vi "SetOscillatorFreq.vi"(8 "error in (no error)":errorcluster, 10 "_oscillator_freq":u32, 11 "PCA in":refnum<class "PCA.lvclass">) -> (0 "error out":errorcluster, 3 "PCA out":refnum<class "PCA.lvclass">)   [LabVIEW 2022 SP3, in "PCA9685.lvlib" / "PCA.lvclass"]
uses:
  PCA.lvclass
  PCA.lvclass/PCA.ctl
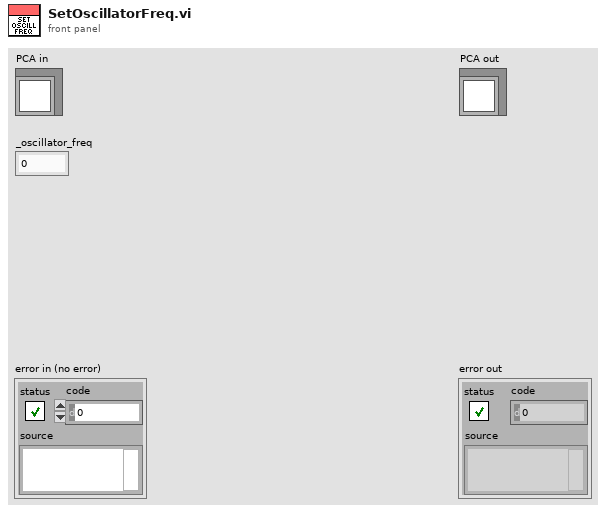
[diagram p1: front panel]
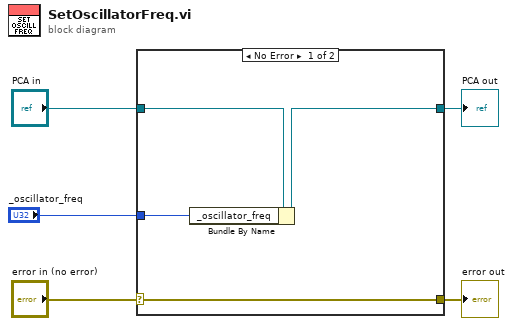
[diagram p0: block diagram]
diagram:
  n1 = case shown="No Error" "error in (no error)" {
    selector: "error in (no error)" -> [w8 w11]
    tunnel: [w8 w11] -> w4
    tunnel: [w7 w10] -> w2
    tunnel: "PCA in" -> [w9 w10]
    tunnel: "_oscillator_freq" -> [w6 _]
    frame No Error {
      n2 = Bundle By Name(cluster=w9, "_oscillator_freq"=w6) -> (w7:refnum<class "PCA.lvclass">)
    }
    frame Error {
    }
  }
  "error out" <- w4
  "PCA out" <- w2
